vi "GSIOC connect.vi"(8 "error in (no error)":errorcluster, 10 "ID (1)":u8=1, 11 "VISA resource name":refnum<visa-resource-name>="COM1") -> (0 "error out":errorcluster, 1 "Connected":bool, 2 "ID out":u8=1, 3 "VISA resource name":refnum<visa-resource-name>)   [LabVIEW 2015]
panel:
  out "error out 2":errorcluster
  out "read buffer":string
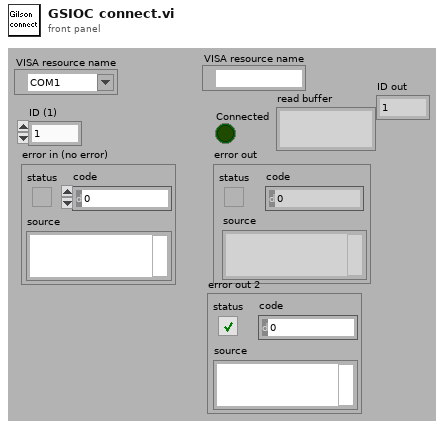
[diagram p1: front panel]
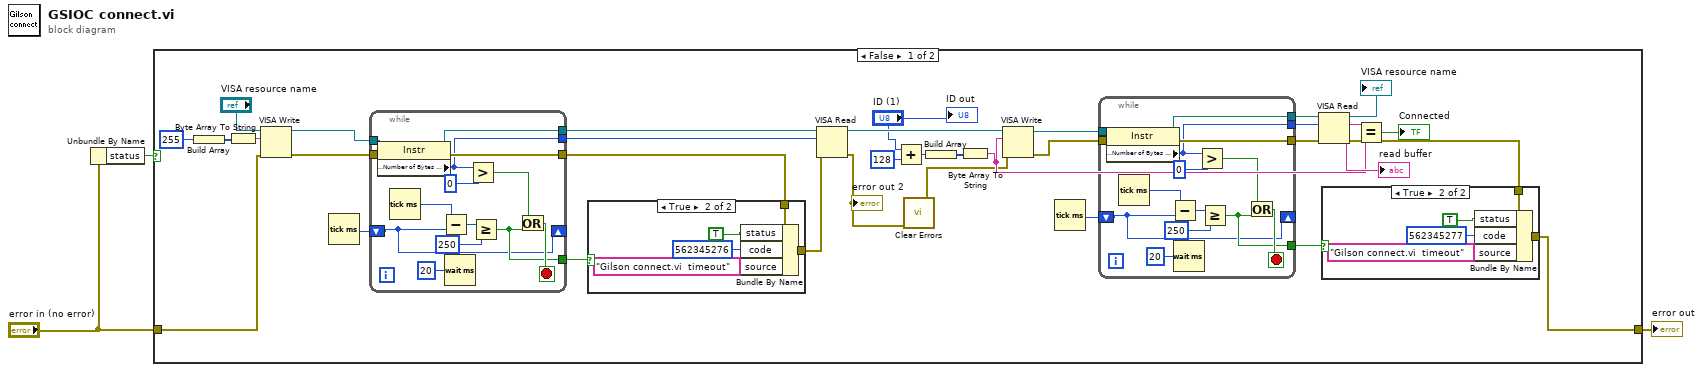
[diagram p0: block diagram]
diagram:
  n1 = Unbundle By Name("error in (no error)") -> ("status"=w3:bool)
  n2 = case shown="False" w3 {
    tunnel: "error in (no error)" -> [w35 w77]
    tunnel: [w34 w77] -> w1
    frame False {
      n3 = Build Array(u8 255) -> (w29:u8[])
      n4 = Byte Array To String(unsigned byte array=w29) -> (string=w28:string)
      n5 = VISA Write(VISA resource name="VISA resource name", write buffer=w28, error in (no error)=w35) -> (VISA resource name out=w32:refnum<visa-resource-name>, error out=w31:errorcluster)  [unwired: 1 out]
      n6 = Tick Count (ms)() -> (millisecond timer value=w26:u32)
      n7 = while {
        tunnel: [w76] -> w9
        tunnel: w31 -> [w75]
        tunnel: [w74] -> w27
        tunnel: [w70] -> w25
        tunnel: [w65] -> w10
        tunnel: w32 -> [w64]
        shift-right: [w63] -> _
        shift-left: w26 -> [w63]
        stop <- w66 stop-if-true
        n8 = property class="Instr"(reference=w64, error in=w75) -> (reference out=w74:refnum<visa-resource-name>, error out=w76:errorcluster, "Serial Settings:Number of Bytes at Serial Port"=w70:u32)
        n9 = Tick Count (ms)() -> (millisecond timer value=w71:u32)
        n10 = Subtract(x=w71, y=w63) -> (x-y=w73:u32)
        n11 = Wait (ms)(milliseconds to wait=u32 20) -> ()  [unwired: 1 out]
        n12 = Greater?(x=w70, y=u32 0) -> (0:w67:bool)
        n13 = Greater Or Equal?(x=w73, y=u32 250) -> (x >= y?=w65:bool)
        n14 = Or(x=w67, y=w65) -> (x .or. y?=w66:bool)
      }
      n15 = case shown="True" w10 {
        tunnel: w9 -> [w37 w42]
        tunnel: [w37 w38] -> w8
        frame False {
        }
        frame True {
          n16 = Bundle By Name(cluster=w42, "status"=TRUE, "code"=562345276, "source"="Gilson connect.vi  timeout") -> (w38:errorcluster)
        }
      }
      n17 = VISA Read(VISA resource name=w27, byte count=w25, error in (no error)=w8) -> (VISA resource name out=w33:refnum<visa-resource-name>, error out=w6:errorcluster)  [unwired: 2 out]
      "error out 2" <- w6
      n18 = Add(x="ID (1)", y=u8 128) -> (x+y=w22:u8)
      n19 = call <vilib>:"Clear Errors.vi"("error in (no error)"=w6) -> ("error out"=w5:errorcluster)  [unwired: 5 in, 1 out]
      n20 = Build Array(w22) -> (w23:u8[])
      n21 = Byte Array To String(unsigned byte array=w23) -> (string=w7:string)
      n22 = VISA Write(VISA resource name=w33, write buffer=w7, error in (no error)=w5) -> (VISA resource name out=w16:refnum<visa-resource-name>, error out=w15:errorcluster)  [unwired: 1 out]
      n23 = Tick Count (ms)() -> (millisecond timer value=w11:u32)
      n24 = while {
        tunnel: [w62] -> w17
        tunnel: w15 -> [w61]
        tunnel: [w60] -> w19
        tunnel: [w56] -> w18
        tunnel: [w51] -> w12
        tunnel: w16 -> [w50]
        shift-right: [w49] -> _
        shift-left: w11 -> [w49]
        stop <- w52 stop-if-true
        n25 = property class="Instr"(reference=w50, error in=w61) -> (reference out=w60:refnum<visa-resource-name>, error out=w62:errorcluster, "Serial Settings:Number of Bytes at Serial Port"=w56:u32)
        n26 = Tick Count (ms)() -> (millisecond timer value=w57:u32)
        n27 = Subtract(x=w57, y=w49) -> (x-y=w59:u32)
        n28 = Wait (ms)(milliseconds to wait=u32 20) -> ()  [unwired: 1 out]
        n29 = Greater?(x=w56, y=u32 0) -> (0:w53:bool)
        n30 = Greater Or Equal?(x=w59, y=u32 250) -> (x >= y?=w51:bool)
        n31 = Or(x=w53, y=w51) -> (x .or. y?=w52:bool)
      }
      n32 = VISA Read(VISA resource name=w19, byte count=w18, error in (no error)=w17) -> (VISA resource name out=→"VISA resource name":refnum<visa-resource-name>, read buffer=w21:string, error out=w14:errorcluster)  [unwired: 1 out]
      "read buffer" <- w21
      n33 = case shown="True" w12 {
        tunnel: w14 -> [w43 w48]
        tunnel: [w43 w44] -> w34
        frame False {
        }
        frame True {
          n34 = Bundle By Name(cluster=w48, "status"=TRUE, "code"=562345277, "source"="Gilson connect.vi  timeout") -> (w44:errorcluster)
        }
      }
      n35 = Equal?(x=w21, y=w7) -> (x = y?=→"Connected":bool)
      "ID out" <- "ID (1)"
    }
    frame True {
    }
  }
  "error out" <- w1
